vi "cmc_Kitchen-Timer.vi"() -> ()   [LabVIEW 2013]
panel:
  in  "Sound Path":path
  in  "stop":bool
  in  "Time (sec)":u8(knob) max=60 step=10 scale=0.0..60.0
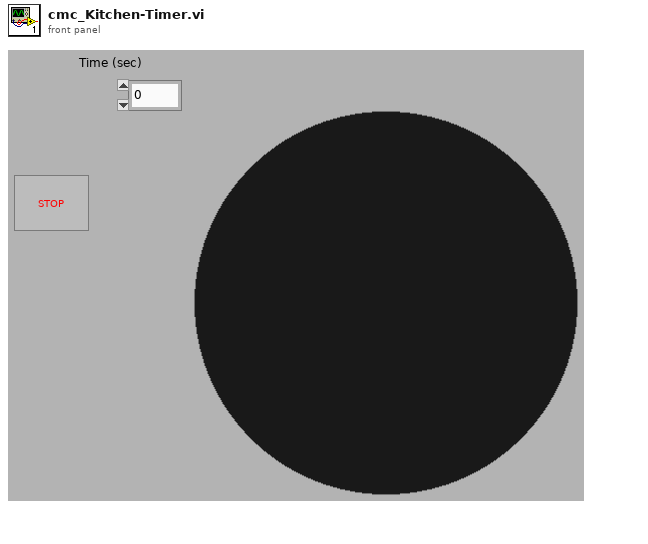
[diagram p1: front panel]
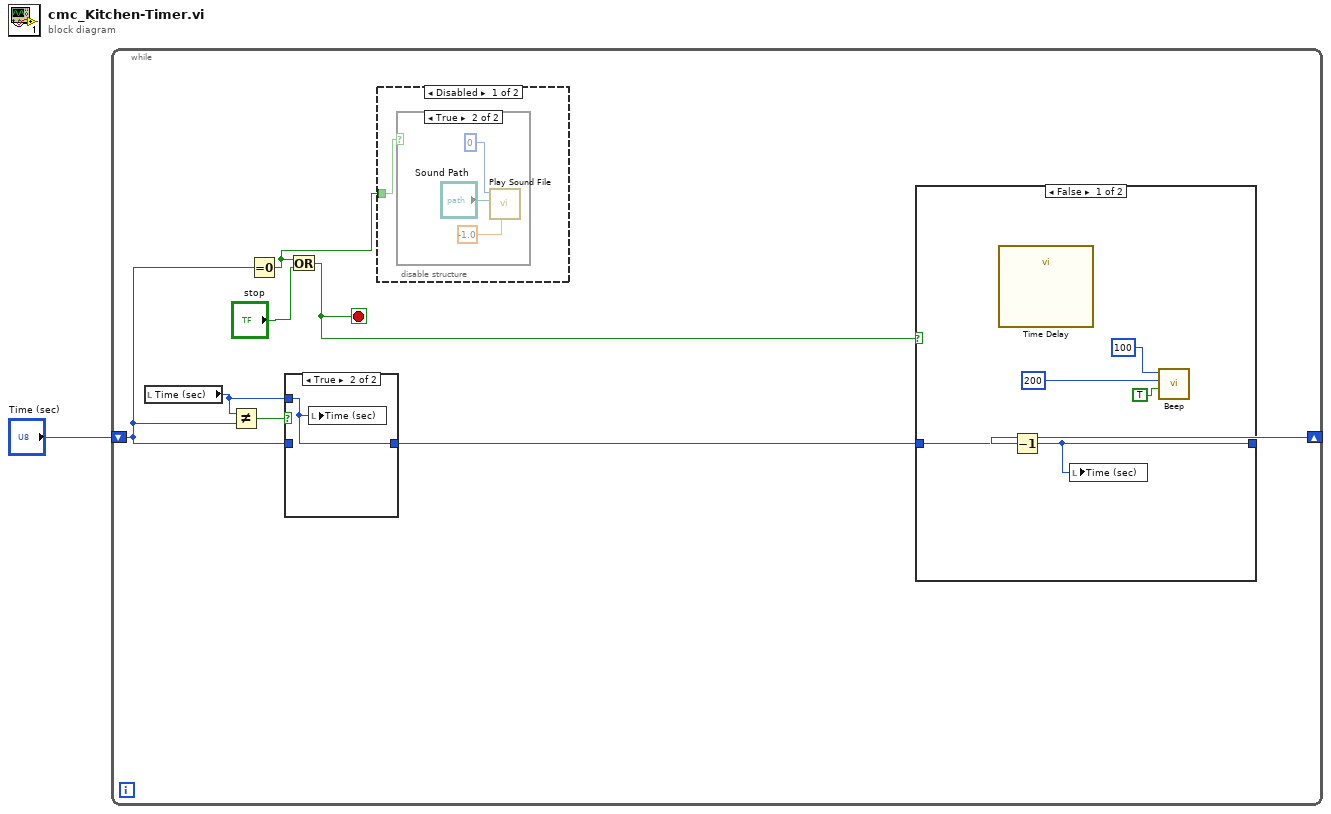
[diagram p0: block diagram]
diagram:
  n1 = while {
    shift-right: [w9] -> _
    shift-left: "Time (sec)" -> [w5]
    stop <- w4 stop-if-true
    n2 = local read "Time (sec)"() -> (w7:u8)
    n3 = Not Equal?(x=w7, y=w5) -> (x != y?=w8:bool)
    n4 = Equal To 0?(x=w5) -> (x = 0?=w3:bool)
    n5 = case shown="True" w8 {
      tunnel: w7 -> [_ w15]
      tunnel: [w14 w15] -> w6
      tunnel: w5 -> [w14 _]
      frame False {
      }
      frame True {
        n6 = local write "Time (sec)"(w15) -> ()
      }
    }
    n7 = Or(x=w3, y="stop") -> (x .or. y?=w4:bool)
    n8 = disable-structure shown="Disabled" {
      disable-tunnel: w3 -> [w10 _]
      frame Disabled {
        n9 = case shown="True" w10 {
          frame False {
          }
          frame True {
            n10 = call <vilib>:"Play Sound File.vi"("timeout (sec)"=-1.0, "path"="Sound Path", "device ID"=u32 0) -> ()  [unwired: 7 in, 2 out]
          }
        }
      }
      frame Enabled {
      }
    }
    n11 = case shown="False" w4 {
      tunnel: [w19 w21] -> w9
      tunnel: w6 -> [w20 w21]
      frame False {
        n12 = call "Time Delay"() -> ()  [unwired: 11 in, 1 out]
        n13 = Decrement(x=w20) -> (x-1=w19:u8)
        n14 = local write "Time (sec)"(w19) -> ()
        n15 = call <vilib>:"Beep.vi"("use system alert? (T)"=TRUE, "duration (msec)"=u32 200, "frequency (Hz)"=u32 100) -> ()  [unwired: 9 in]
      }
      frame True {
      }
    }
  }
